vi "CRYCheck String Array Equal.vi"(11 "In Array":string[](array[string])) -> (2 "Equal":bool, 3 "Name String":string)   [LabVIEW 2013]
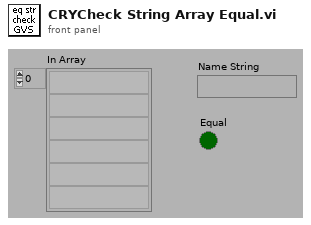
[diagram p1: front panel]
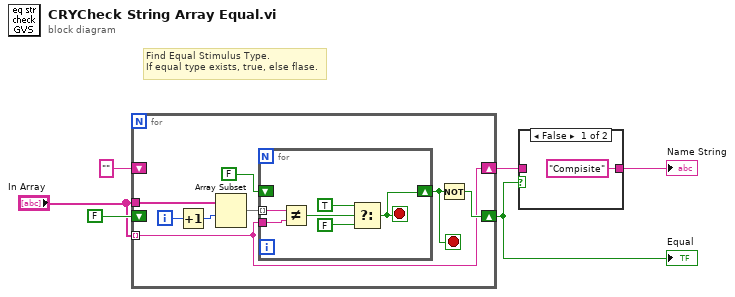
[diagram p0: block diagram]
diagram:
  # "Find Equal Stimulus Type.\nIf equal type exists, true, else flase."
  n1 = for {
    tunnel: "In Array" -> [w9] mode=indexing
    tunnel: "In Array" -> [w12]
    shift-right: [w9] -> w2
    shift-left: "" ("Type Name") -> [_]
    shift-right: [w13] -> w3
    shift-left: FALSE -> [_]
    i -> [w14]
    stop <- w8 stop-if-true
    n2 = Increment(x=w14) -> (x+1=w11:i32)
    n3 = Array Subset(array=w12, index=w11) -> (w10:string[])  [unwired: 1 in]
    n4 = for {
      tunnel: w10 -> [w18] mode=indexing
      tunnel: w9 -> [w17]
      shift-right: [w15] -> w8
      shift-left: FALSE -> [_]
      stop <- w15 stop-if-true
      n5 = Not Equal?(x=w18, y=w17) -> (x != y?=w16:bool)
      n6 = Select(t=TRUE, s=w16, f=FALSE) -> (s? t:f=w15:bool)
    }
    n7 = Not(x=w8) -> (.not. x?=w13:bool)
  }
  "Equal" <- w3
  n8 = case shown="False" w3 {
    tunnel: ["Compisite" ("Type Name") w22] -> w1
    tunnel: w2 -> [_ w22]
    frame False {
    }
    frame True {
    }
  }
  "Name String" <- w1
